vi "Delete Queue.vi"(8 "error in (no error)":errorcluster, 11 "SQS":refnum<class "NI_AWS_SQS.lvclass">) -> (0 "error out":errorcluster)   [LabVIEW 2015, in "NI_AWS_SQS.lvclass"]
uses:
  NI_AWS_SQS.lvclass
  Core/Request Options.ctl
  Core/Name Value Pair.ctl
  NI_AWS_SQS.lvclass/NI_AWS_SQS.ctl
  Read Account Number.vi
  Read Name.vi
  Core/NI_AWS_Core.lvclass
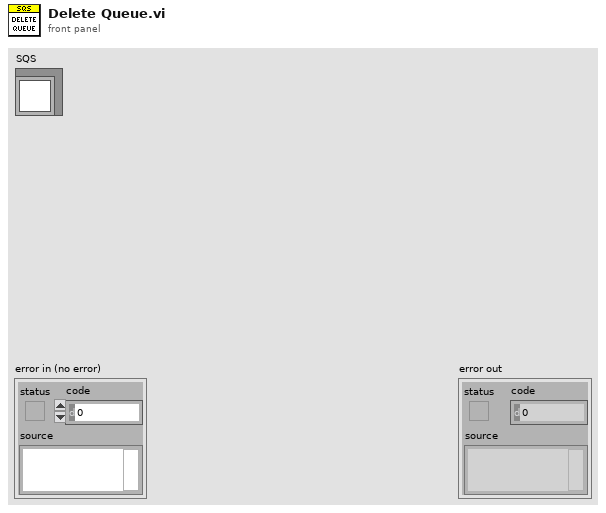
[diagram p1: front panel]
types:
  T1 = typedef "NI_AWS_Core.lvclass/Name Value Pair.ctl" = cluster{"name":string, "value":string}
  T2 = typedef "NI_AWS_Core.lvclass/Request Options.ctl" = cluster{"request headers":T1[], "request parameters":T1[], "request body":string}
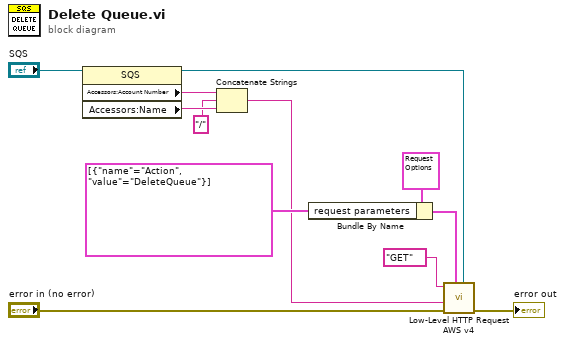
[diagram p0: block diagram]
diagram:
  n1 = property class="SQS"(reference="SQS") -> (reference out=w2:refnum<class "NI_AWS_SQS.lvclass">, "Accessors:Account Number"=w6:string, "Accessors:Name"=w5:string)  [unwired: 1 in, 1 out]
  n2 = Concatenate Strings(w6, "/", w5) -> (w1:string)
  n3 = Bundle By Name(cluster=T2 {"request headers"=[], "request parameters"=[{"name"="Action", "value"="ListQueues"}], "request body"=""} ("Request Options"), "request parameters"=T1[] [{"name"="Action", "value"="DeleteQueue"}]) -> (w10:T2)
  n4 = call "Low-Level HTTP Request AWS v4.vi"("AWS Core"=w2, "Request Options"=w10, "error in (no error)"="error in (no error)", "URL Suffix"=w1, "HTTP-Verb"="GET") -> ("error out"=→"error out":errorcluster)  [unwired: 4 in, 2 out]
